vi "CMTracker.vi"(11 "BodyID":dbl=3.0) -> (3 "CMTrackData":T1)   [LabVIEW 2020]
panel:
  in  "VrpnServer":string="MCServer@169.254.0.5"
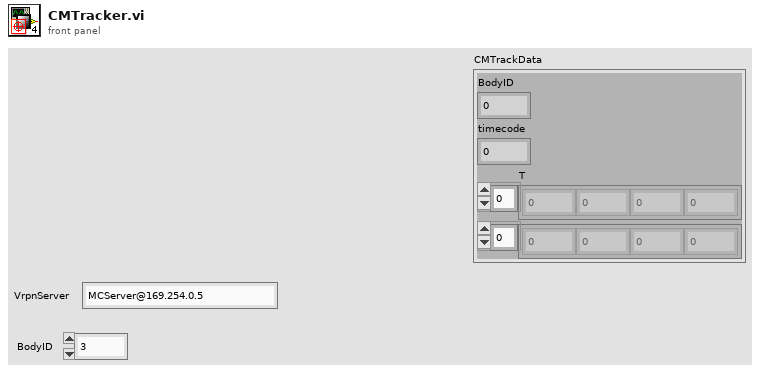
[diagram p1: front panel]
types:
  T1 = cluster{"BodyID":i32, "timecode":i32, "T":dbl[], dbl[]}
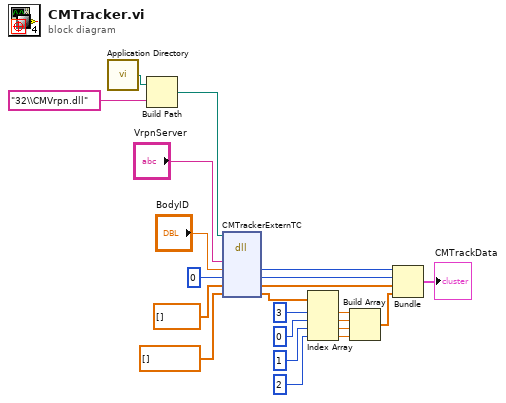
[diagram p0: block diagram]
diagram:
  n1 = call <vilib>:"Application Directory.vi"() -> ("Application Directory"=w22:path)
  n2 = Build Path(base path=w22, name or relative path="32\\CMVrpn.dll") -> (appended path=w21:path)
  n3 = dll-call lib="C" fn="CMTrackerExternTC"(path in=w21, "VrpnServer"="VrpnServer", "BodyID"="BodyID", "timecode"=0, "T"=dbl[] [], "R_Quat"=dbl[] []) -> ("BodyID"=w5:i32, "timecode"=w4:i32, "T"=w3:dbl[], "R_Quat"=w14:dbl[])  [unwired: 4 in, 2 out]
  n4 = Index Array(array=w14, index #1=3, index #2=0, index #3=1, index #4=2) -> (element #1=w9:dbl, element #2=w8:dbl, element #3=w7:dbl, element #4=w6:dbl)
  n5 = Build Array(w9, w8, w7, w6) -> (w2:dbl[])
  n6 = Bundle("BodyID"=w5, "timecode"=w4, "T"=w3, w2) -> (→"CMTrackData":T1)  [unwired: 1 in]
